vi "two_button.vi"() -> ()   [LabVIEW 2023, in "task_1.lvlib"]
uses:
  task_1.lvlib
  C:/Windows/System32/user32.dll
panel:
  out "error out":errorcluster
  in  "error in (no error)":errorcluster
  out "button_b_out":bool
  out "button_a_out":bool
  in  "button_b":bool
  in  "button_a":bool
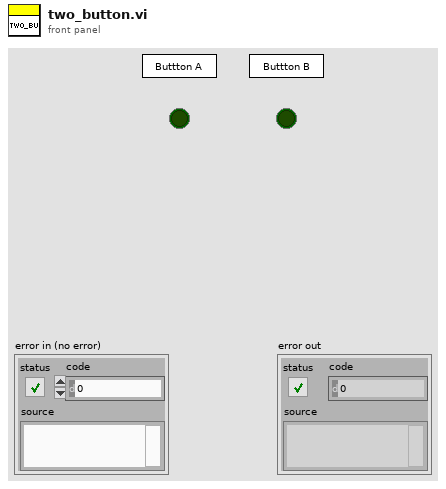
[diagram p1: front panel]
types:
  T1 = typedef "LVPositionTypeDef.ctl" = cluster{"Left":i32, "Top":i32}
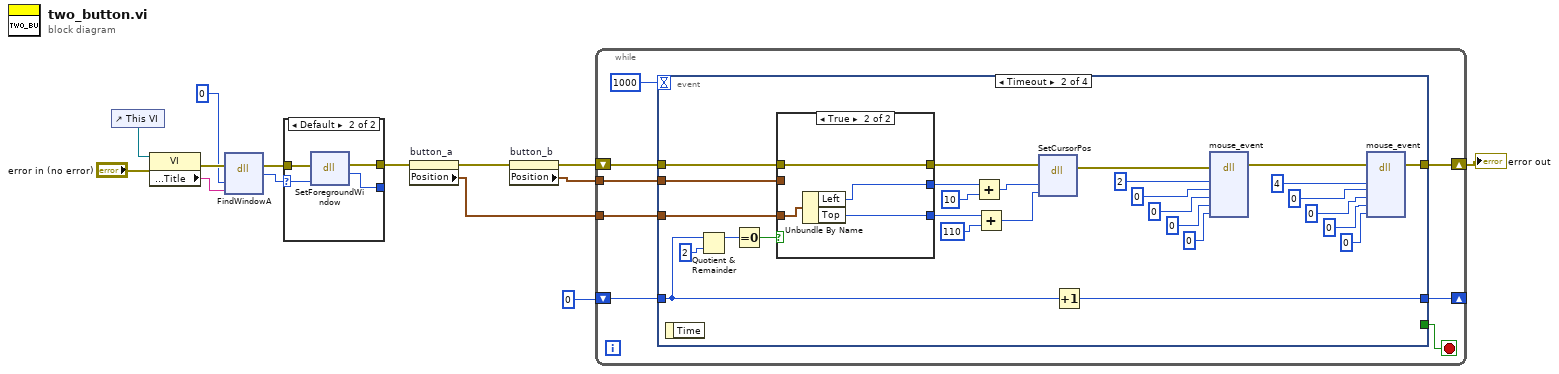
[diagram p0: block diagram]
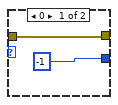
[diagram p2: hidden frame]
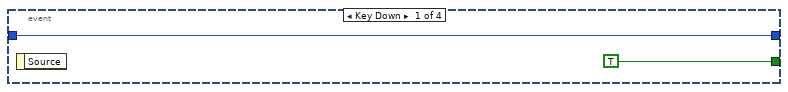
[diagram p3: hidden frame]
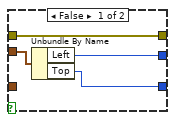
[diagram p4: hidden frame]
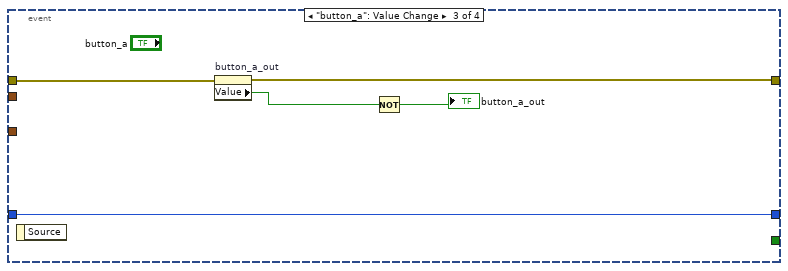
[diagram p5: hidden frame]
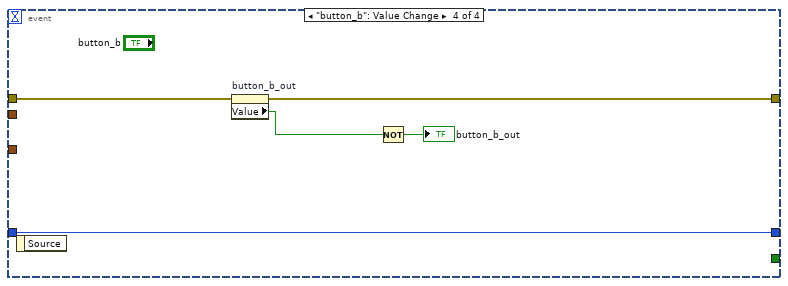
[diagram p6: hidden frame]
diagram:
  n1 = control-ref of="This VI"() -> (w14:refnum<vi>)
  n2 = property class="VI"(reference=w14, error in="error in (no error)") -> (error out=w11:errorcluster, "Front Panel.Title"=w12:string)  [unwired: 1 out]
  n3 = dll-call lib="C:/Windows/System32/user32.dll" fn="FindWindowA"(error in=w11, "lpClassName"=0, "lpWindoeName"=w12) -> (error out=w9:errorcluster, "HWND"=w8:u64)  [unwired: 4 in, 1 out]
  n4 = case shown="Default" w8 {
    selector: w8 -> [_ w20]
    tunnel: w9 -> [w15 w19]
    tunnel: [-1 ("Bool") w18] -> _
    tunnel: [w15 w17] -> w7
    frame 0 {
    }
    frame Default {
      n5 = dll-call lib="C:/Windows/System32/user32.dll" fn="SetForegroundWindow"(error in=w19, "HWND"=w20) -> (error out=w17:errorcluster, "Bool"=w18:i32)  [unwired: 3 in, 1 out]
    }
  }
  n6 = property on="button_a" class="Bool"(error in=w7) -> (error out=w6:errorcluster, "Position"=w4:T1)  [unwired: 1 in, 1 out]
  n7 = property on="button_b" class="Bool"(error in=w6) -> (error out=w3:errorcluster, "Position"=w5:T1)  [unwired: 1 in, 1 out]
  n8 = while {
    tunnel: w5 -> [w26]
    tunnel: w4 -> [w25]
    shift-right: [w23] -> w2
    shift-left: w3 -> [w24]
    shift-right: [w21] -> _
    shift-left: 0 -> [w22]
    stop <- w27 stop-if-true
    n9 = event shown="[1] Timeout" {
      selector: _ -> [_ _ _ _]
      dyn-events: _ -> [_ _ _ _]
      timeout: 1000 -> [_ _ _ _]
      tunnel: [TRUE _ _ _] -> w27
      tunnel: w26 -> [_ w42 _ _]
      tunnel: w25 -> [_ w41 _ _]
      tunnel: w24 -> [_ w36 w69 w74]
      tunnel: [_ w43 w68 w73] -> w23
      tunnel: w22 -> [w29 w32 w67 w72]
      tunnel: [w29 w35 w67 w72] -> w21
      event Key Down {
        n10 = event-data() -> ()  [unwired: 1 in, 1 out]
      }
      event Timeout {
        n11 = event-data() -> ()  [unwired: 1 in, 1 out]
        n12 = Quotient & Remainder(x=w32, y=2) -> (x-y*floor(x/y)=w34:i32)  [unwired: 1 out]
        n13 = Equal To 0?(x=w34) -> (x = 0?=w33:bool)
        n14 = case shown="True" w33 {
          tunnel: w36 -> [w62 w65]
          tunnel: w42 -> [w61 _]
          tunnel: w41 -> [_ w66]
          tunnel: [w62 w65] -> w56
          tunnel: [w60 w64] -> w55
          tunnel: [w59 w63] -> w54
          frame False {
            n15 = Unbundle By Name(w61) -> ("Left"=w60:i32, "Top"=w59:i32)
          }
          frame True {
            n16 = Unbundle By Name(w66) -> ("Left"=w64:i32, "Top"=w63:i32)
          }
        }
        n17 = Add(x=w55, y=10) -> (x+y=w40:i32)
        n18 = Add(x=w54, y=110) -> (x+y=w39:i32)
        n19 = dll-call lib="C:/Windows/System32/user32.dll" fn="SetCursorPos"(error in=w56, "X"=w40, "Y"=w39) -> (error out=w57:errorcluster)  [unwired: 5 in, 1 out]
        n20 = Increment(x=w32) -> (x+1=w35:i32)
        n21 = dll-call lib="C:/Windows/System32/user32.dll" fn="mouse_event"(error in=w57, "flag"=u32 2, "dx"=u32 0, "dy"=u32 0, "dwData"=u32 0, "dwExtra"=u32 0) -> (error out=w58:errorcluster)  [unwired: 8 in, 1 out]
        n22 = dll-call lib="C:/Windows/System32/user32.dll" fn="mouse_event"(error in=w58, "flag"=u32 4, "dx"=u32 0, "dy"=u32 0, "dwData"=u32 0, "dwExtra"=u32 0) -> (error out=w43:errorcluster)  [unwired: 8 in, 1 out]
      }
      event "button_a": Value Change {
        n23 = event-data() -> ()  [unwired: 1 in, 1 out]
        n24 = property on="button_a_out" class="Bool (strict)"(error in=w69) -> (error out=w68:errorcluster, "Value"=w71:bool)  [unwired: 1 in, 1 out]
        n25 = Not(x=w71) -> (.not. x?=→"button_a_out":bool)
      }
      event "button_b": Value Change {
        n26 = event-data() -> ()  [unwired: 1 in, 1 out]
        n27 = property on="button_b_out" class="Bool (strict)"(error in=w74) -> (error out=w73:errorcluster, "Value"=w76:bool)  [unwired: 1 in, 1 out]
        n28 = Not(x=w76) -> (.not. x?=→"button_b_out":bool)
      }
    }
  }
  "error out" <- w2
